vi "ctn.vi"(6 "x":dbl, 7 "Numérique en entrée":dbl, 9 "valeur par défaut (0 I32)":dbl, 10 "String from arduino":string, 11 "utiliser le séparateur décimal du système (V)":bool) -> (3 "Numérique en sortie":dbl)   [LabVIEW 2020]
uses:
  Variables globales outil isospi sans MCU.vi
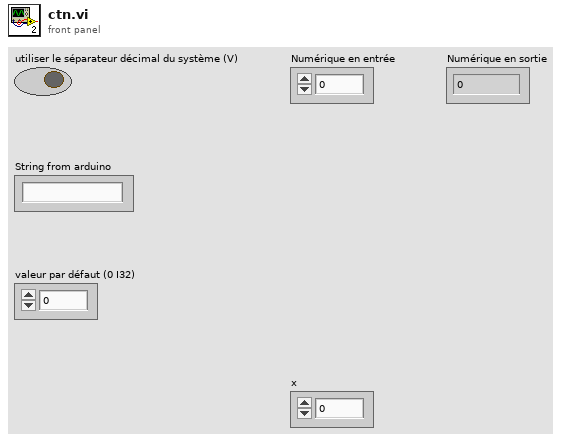
[diagram p1: front panel]
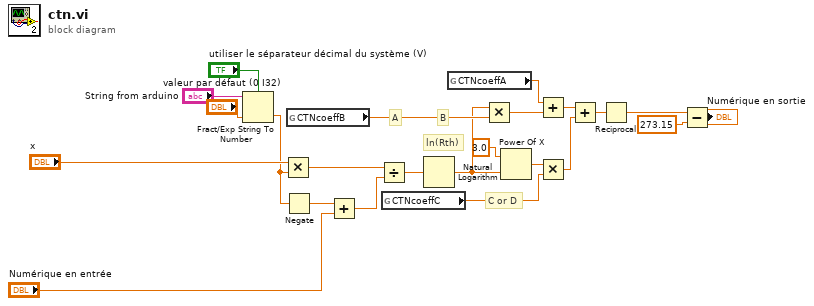
[diagram p0: block diagram]
diagram:
  # "C or D"
  # "B"
  # "ln(Rth)"
  # "A"
  n1 = Fract/Exp String To Number(use system decimal point (T)="utiliser le séparateur décimal du système (V)", string="String from arduino", default (0 dbl)="valeur par défaut (0 I32)") -> (number=w18:dbl)  [unwired: 1 in, 1 out]
  n2 = Multiply(x="x", y=w18) -> (x*y=w10:dbl)
  n3 = Negate(x=w18) -> (-x=w8:dbl)
  n4 = global read "Variables globales outil isospi sans MCU.vi" "CTNcoeffB"() -> (w22:dbl)
  n5 = Add(x=w8, y="Numérique en entrée") -> (x+y=w11:dbl)
  n6 = Divide(x=w10, y=w11) -> (x/y=w9:dbl)
  n7 = global read "Variables globales outil isospi sans MCU.vi" "CTNcoeffC"() -> (w23:dbl)
  n8 = Natural Logarithm(1:w9) -> (0:w3:dbl)
  n9 = global read "Variables globales outil isospi sans MCU.vi" "CTNcoeffA"() -> (w21:dbl)
  n10 = Multiply(x=w3, y=w22) -> (x*y=w1:dbl)
  n11 = Power Of X(1:w3, 2:3.0 ("y")) -> (0:w4:dbl)
  n12 = Add(x=w21, y=w1) -> (x+y=w5:dbl)
  n13 = Multiply(x=w4, y=w23) -> (x*y=w6:dbl)
  n14 = Add(x=w5, y=w6) -> (x+y=w7:dbl)
  n15 = Reciprocal(x=w7) -> (1/x=w12:dbl)
  n16 = Subtract(x=w12, y=273.15) -> (x-y=→"Numérique en sortie":dbl)
